vi "Wait on Multiple Notifiers.vi"() -> ()   [LabVIEW 2023]
doc: "This VI demonstrates the use and behavior of the Wait on Notification from Multiple function, which allows a single part of a diagram to wait for notifiers that you specify. This function returns an array of the data values that the notifications receive. If you adjust the delay controls on the front panel of this VI, the Wait on Notification from Multiple function executes on every data point it receives regardless of which Send Notification function sends the data.\n\nThe Send Notification functions pass sine waves in two parallel While loops. The Wait on Notification from Multiple function receives this data in a third While loop, and the Notifications Chart plots the two sine waves. If the <b>Notification Loop Delay</b> is less than <b>Notifier 1 Loop Delay</b> or <b>Notifier 2 Loop Delay</b>, the Wait on Notification from Multiple function continues to execute as long as it receives one of the notifications."
panel:
  out "Notifications Chart":cluster{"[0]":dbl, "[1]":dbl}(graph)
  in  "Notification Loop Delay (ms)":u32=200 step=10
  in  "Notifier 2 Loop Delay (ms)":u32=100 step=10
  in  "Notifier 1 Loop Delay (ms)":u32=50 step=10
  in  "Stop":bool
  # "Overview: Demonstrates the use of the Wait on Notification from Multiple function.\nInstructions:\n1. Run the VI.\n2. Adjust the controls below and observe the behavior of the notification plots.\n3. Set the Notification Loop Delay to less than one or both of the other delays and observe that erroneous values are displayed.\n4. Click Stop to stop the VI."
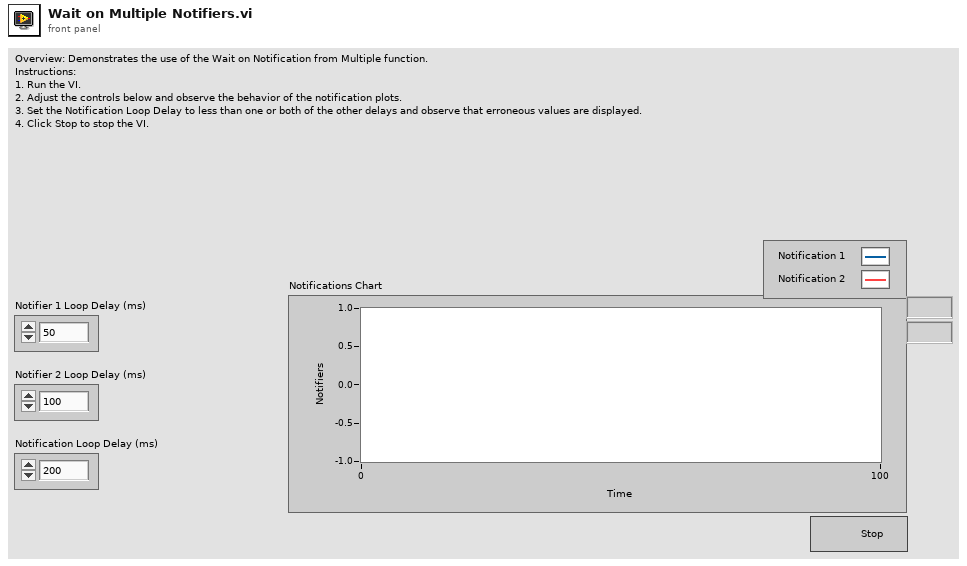
[diagram p1: front panel]
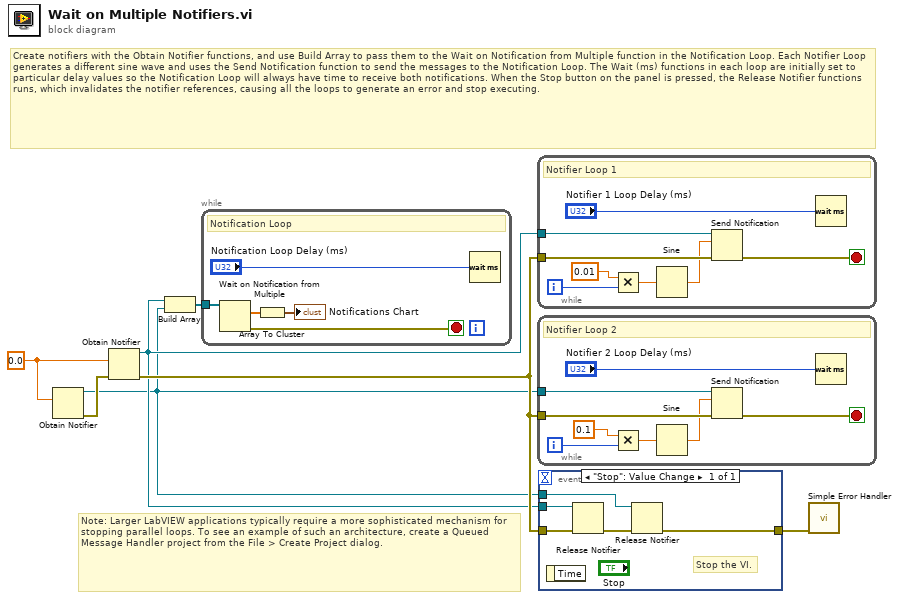
[diagram p0: block diagram]
diagram:
  w6 = 0.0
  # "Note: Larger LabVIEW applications typically require a more sophisticated mechanism for stopping parallel loops. To see an example of such an architecture, create a Queued Message Handler project from the File > Create Project dialog."
  # "Create notifiers with the Obtain Notifier functions, and use Build Array to pass them to the Wait on Notification from Multiple function in the Notification Loop. Each Notifier Loop generates a different sine wave and uses the Send Notification function to send the messages to the Notification Loop. The Wait (ms) functions in each loop are initially set to particular delay values so the Notification Loop will always have time to receive both notifications. When the Stop button on the panel is pressed, the Release Notifier functions runs, which invalidates the notifier references, causing all the loops to generate an error and stop executing."
  n1 = Obtain Notifier(notification data type=w6) -> (notifier out=w2:refnum<notifier>, error out=w5:errorcluster)  [unwired: 3 in, 1 out]
  n2 = Obtain Notifier(notification data type=w6, error in (no error)=w5) -> (notifier out=w3:refnum<notifier>, error out=w4:errorcluster)  [unwired: 2 in, 1 out]
  n3 = Build Array(w3, w2) -> (w7:refnum<notifier>[])
  n4 = while {
    tunnel: w7 -> [w12]
    stop <- w8 stop-if-true
    # "Notification Loop"
    n5 = Wait on Notification from Multiple(0:w12) -> (9:w10:dbl[], 11:w8:errorcluster)  [unwired: 2 in, 3 out]
    n6 = Array To Cluster(array=w10) -> (cluster=→"Notifications Chart":cluster{"[0]":dbl, "[1]":dbl})
    n7 = Wait (ms)(milliseconds to wait="Notification Loop Delay (ms)") -> ()  [unwired: 1 out]
  }
  n8 = while {
    tunnel: w3 -> [w20]
    tunnel: w4 -> [w19]
    i -> [w14]
    stop <- w15 stop-if-true
    # "Notifier Loop 1"
    n9 = Multiply(x=0.01, y=w14) -> (x*y=w17:dbl)
    n10 = Sine(x=w17) -> (sin(x)=w16:dbl)
    n11 = Send Notification(notification=w16, notifier=w20, error in (no error)=w19) -> (error out=w15:errorcluster)  [unwired: 1 out]
    n12 = Wait (ms)(milliseconds to wait="Notifier 1 Loop Delay (ms)") -> ()  [unwired: 1 out]
  }
  n13 = while {
    tunnel: w2 -> [w28]
    tunnel: w4 -> [w27]
    i -> [w22]
    stop <- w23 stop-if-true
    # "Notifier Loop 2"
    n14 = Multiply(x=0.1, y=w22) -> (x*y=w25:dbl)
    n15 = Sine(x=w25) -> (sin(x)=w24:dbl)
    n16 = Send Notification(notification=w24, notifier=w28, error in (no error)=w27) -> (error out=w23:errorcluster)  [unwired: 1 out]
    n17 = Wait (ms)(milliseconds to wait="Notifier 2 Loop Delay (ms)") -> ()  [unwired: 1 out]
  }
  n18 = event shown="[0] \"Stop\": Value Change" {
    selector: _ -> [_]
    dyn-events: _ -> [_]
    timeout: _ -> [_]
    tunnel: w4 -> [w33]
    tunnel: w3 -> [w32]
    tunnel: w2 -> [w30]
    tunnel: [w29] -> w1
    event "Stop": Value Change {
      # "Stop the VI."
      n19 = event-data() -> ()  [unwired: 1 in, 1 out]
      n20 = Release Notifier(notifier=w32, error in (no error)=w33) -> (error out=w31:errorcluster)  [unwired: 1 in, 2 out]
      n21 = Release Notifier(notifier=w30, error in (no error)=w31) -> (error out=w29:errorcluster)  [unwired: 1 in, 2 out]
    }
  }
  n22 = call <vilib>:"Simple Error Handler.vi"("error in (no error)"=w1) -> ()  [unwired: 1 in, 8 out]
